vi "RegReadConfigName.vi"(8 "errorIN":errorcluster, 10 "ConfigName_Ref":refnum<vi>) -> (0 "error out":errorcluster, 2 "ConfigName":string)   [LabVIEW 2010]
uses:
  <vilib>/registry/registry.llb/Registry RtKey.ctl
  <vilib>/registry/registry.llb/Registry SAM.ctl
  <vilib>/registry/registry.llb/Read Registry Value Simple STR.vi
  <vilib>/registry/registry.llb/Write Registry Value Simple STR.vi
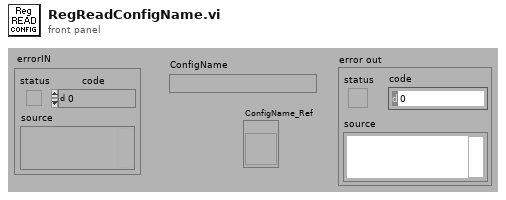
[diagram p1: front panel]
types:
  T1 = enum32{"REG_OPTION_NON_VOLATILE", "REG_OPTION_VOLATILE", "REG_OPTION_BACKUP_RESTORE"}
  T2 = typedef "Registry RtKey.ctl" = enum32{"HKEY_CLASSES_ROOT", "HKEY_CURRENT_USER", "HKEY_LOCAL_MACHINE", "HKEY_USERS", "HKEY_PERFORMANCE_DATA", "HKEY_CURRENT_CONFIG", "HKEY_DYN_DATA"}
  T3 = typedef "Registry SAM.ctl" = enum32{"KEY_QUERY_VALUE", "KEY_SET_VALUE", "KEY_CREATE_SUB_KEY", "KEY_ENUMERATE_SUB_KEYS", "KEY_NOTIFY", "KEY_CREATE_LINK", "KEY_READ", "KEY_WRITE", "KEY_ALL_ACCESS", "KEY_READ | KEY_WRITE"}
  T4 = typedef "Registry refnum.ctl" = refnum<k1>
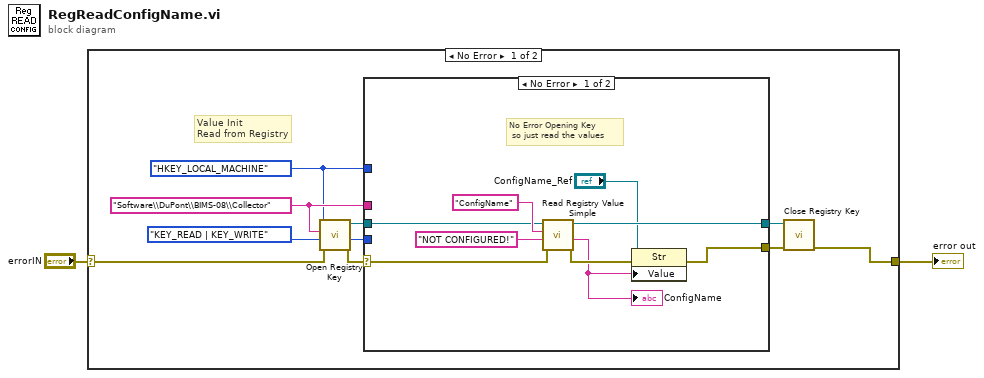
[diagram p0: block diagram]
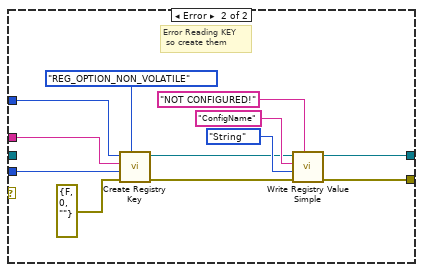
[diagram p2: hidden frame]
diagram:
  n1 = case shown="No Error" "errorIN" {
    selector: "errorIN" -> [w3 w33]
    tunnel: [w4 w33] -> w2
    frame No Error {
      w10 = Registry_RtKey."HKEY_LOCAL_MACHINE" ("root key (HKEY_LOCAL_MACHINE)")
      w9 = Registry_SAM."KEY_READ | KEY_WRITE" ("security access mask (KEY_READ | KEY_WRITE)")
      w11 = "Software\\DuPont\\BIMS-08\\Collector" ("subkey")
      # "Value Init\nRead from Registry"
      n2 = call <vilib>:"Open Registry Key.vi"("error in (no error)"=w3, "security access mask (KEY_READ | KEY_WRITE)"=w9, "subkey"=w11, "root key (HKEY_LOCAL_MACHINE)"=w10) -> ("error out"=w7:errorcluster, "refnum out"=w8:T4)  [unwired: 6 out]
      n3 = case shown="No Error" w7 {
        selector: w7 -> [w14 _]
        tunnel: w8 -> [w15 _]
        tunnel: [w17 w27] -> w6
        tunnel: [w18 w26] -> w5
        tunnel: w9 -> [_ w32]
        tunnel: w11 -> [_ w31]
        tunnel: w10 -> [_ w30]
        frame No Error {
          # "No Error Opening Key\n so just read the values"
          n4 = call-poly <vilib>:"Read Registry Value Simple.vi"("error in (no error)"=w14, "default data"="NOT CONFIGURED!", "value"="ConfigName", "refnum"=w15) -> ("error out"=w19:errorcluster, "String/Binary data"=w13:string, "refnum out"=w17:T4)  [unwired: 3 out]
          "ConfigName" <- w13
          n5 = property on="Property Node" class="Str"(reference="ConfigName_Ref", error in=w19, "Value"=w13) -> (error out=w18:errorcluster)  [unwired: 1 out]
        }
        frame Error {
          # "Error Reading KEY\n so create them"
          n6 = call <vilib>:"Create Registry Key.vi"("options"=T1."REG_OPTION_NON_VOLATILE", "error in (no error)"=errorcluster {"status"=FALSE, "code"=0, "source"=""}, "security access mask (KEY_READ | KEY_WRITE)"=w32, "subkey"=w31, "root key (HKEY_LOCAL_MACHINE)"=w30) -> ("error out"=w22:errorcluster, "refnum out"=w23:T4)  [unwired: 5 out]
          n7 = call-poly <vilib>:"Write Registry Value Simple.vi"("String/Binary data"="NOT CONFIGURED!" ("default data"), "error in (no error)"=w22, "simple data type"=enum16{"String", "Binary", "DWORD"}."String", "value"="ConfigName", "refnum"=w23) -> ("error out"=w26:errorcluster, "refnum out"=w27:T4)  [unwired: 3 out]
        }
      }
      n8 = call <vilib>:"Close Registry Key.vi"("error in (no error)"=w5, "refnum"=w6) -> ("error out"=w4:errorcluster)  [unwired: 5 out]
    }
    frame Error {
    }
  }
  "error out" <- w2
